vi "DENFPGA.vi"(8 "error in (no error)":errorcluster, 9 "Single shot":bool, 10 "Reads":u8[](array[numeric])=[0, 0, 0, 0, 0, 0, 0, 0, 0, 0, 0, 0, 0, 0, 0, 0, 0, 0, 0, 0, 0, 0, 0, 0, 0, 0, 0, 0, 0, 0, 0, 0, 0, 0, 0, 0, 0, 0, 0, 0, 0, 0, 0, 0, 0, 0, 0, 0, 0, 0, 0, 0, 0, 0, 0, 0, 0, 0, 0, 0, 0, 0, 0, 0, 0, 0, 0, 0, 0, 0, 0, 0, 0, 0, 0, 0, 0, 0, 0, 0, 0, 0, 0, 0, 0, 0, 0, 0, 0, 0, 0, 0, 0, 0, 0, 0, 0, 0, 0, 0], 11 "Commands":u8[](array[numeric])=[0, 0, 0, 0, 0, 0, 0, 0, 0, 0, 0, 0, 0, 0, 0, 0, 0, 0, 0, 0, 0, 0, 0, 0, 0, 0, 0, 0, 0, 0, 0, 0, 0, 0, 0, 0, 0, 0, 0, 0, 0, 0, 0, 0, 0, 0, 0, 0, 0, 0, 0, 0, 0, 0, 0, 0, 0, 0, 0, 0, 0, 0, 0, 0, 0, 0, 0, 0, 0, 0, 0, 0, 0, 0, 0, 0, 0, 0, 0, 0, 0, 0, 0, 0, 0, 0, 0, 0, 0, 0, 0, 0, 0, 0, 0, 0, 0, 0, 0, 0]) -> (0 "error out":errorcluster, 1 "Telemetry":u8[](array[numeric]), 2 "IP on error/exit":i16, 3 "Readouts":u8[](array[numeric]), 4 "code":i32, 5 "status":bool)   [LabVIEW 2018]
uses:
  TestMPU.lvclass
  <vilib>/rvi/Emulation/niFpgaSctlEmulationGetInTimedLoop.vi
  <vilib>/rvi/DataTransferAndStorage/Container/Common/niFpgaContainerGetUniqueNameForEmu.vi
  <vilib>/rvi/DataTransferAndStorage/Container/Common/niFpgaContainerSetEmuInfo.vi
  <vilib>/rvi/eio/common/nirviEmuReportErrorAndStop.vi
  <vilib>/rvi/DataTransferAndStorage/Container/Common/niFpgaContainerExecOnDevCompGetState.vi
  <vilib>/rvi/Emulation/niFpgaEmulationIsFPGAContextNoSignature.vi
  <vilib>/rvi/errors/niFpgaSetErrorForExecOnDevCompSimple.vi
  <vilib>/rvi/FIFO/Fifo_Resource/nirvififoEmulationSetSize.vi
  <vilib>/rvi/FIFO/Fifo_Resource/nirviFifoEmulationQueueMgr.vi
  <instcachedir>/0/nirviFifoEmulationQueueMgr_E5CAEC123FF24DC58D834DCA3CDAA9B5.lvgen/nirviFifoEmulationQueueMgr_E5CAEC123FF24DC58D834DCA3CDAA9B5_001.vi
  <vilib>/rvi/FIFO/Fifo_Resource/nirvififoEmulationDetermineInputValidOut.vi
  <vilib>/rvi/FIFO/Fifo_Resource/nirvififoEmulationCreateLock.vi
  <vilib>/rvi/Emulation/niFpgaProcessEmulError.vi
  <vilib>/rvi/FIFO/Fifo_Resource/nirvififoEmulationObtainLock.vi
  <vilib>/rvi/FIFO/Fifo_Resource/nirvififoEmulationReleaseLock.vi
  <vilib>/rvi/occurrence/nirviWaitOnOccurrenceBase.vi
  <vilib>/rvi/errors/nirviReportUnexpectedCaseInternalError.vi
  <vilib>/rvi/errors/nirviReportUnexpectedCaseInternalError (U32).vi
  <vilib>/Utility/error.llb/Clear Errors.vi
  <vilib>/rvi/interface/RandomDataEmulation/niFpgaRandomDataHandleErrors.vi
  <vilib>/rvi/LocalResourceManager/LocalResourceManager.xnode
  <vilib>/rvi/DataTransferAndStorage/Container/XNode/niFpgaContainer.xnode
  <vilib>/rvi/FIFO/Fifo_Resource/niFpgaFifoEmulationRefIn.vi
panel:
  out "Writes":u8[](array[numeric])
  # "You need to fill in commands. First element of\ncommands is number of commands (same for reads, as \ncommands array is fixed size itself). If number of commands\nis <= 0, error -23 is triggered and execution doesn't proceed."
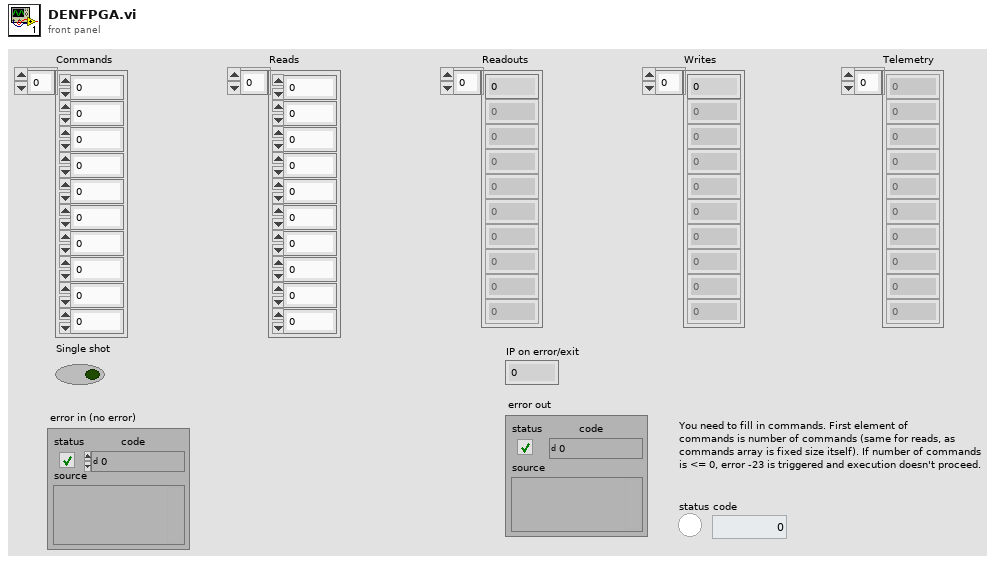
[diagram p1: front panel]
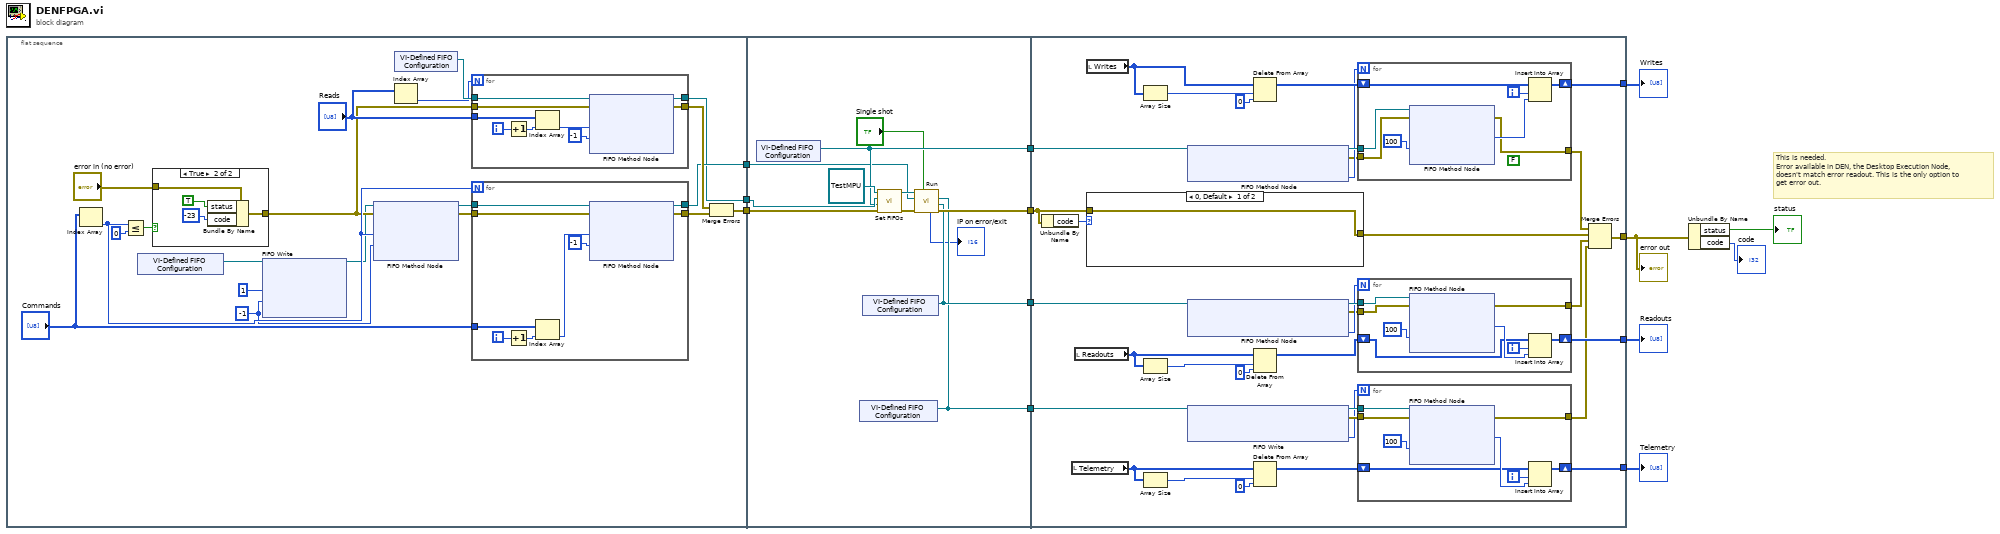
[diagram p0: block diagram]
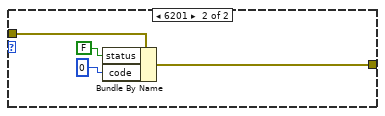
[diagram p3: hidden frame]
diagram:
  # "This is needed.\nError available in DEN, the Desktop Execution Node,\ndoesn't match error readout. This is the only option to \nget error out."
  n1 = flat-sequence {
    tunnel: [w24] -> w13
    tunnel: [w23] -> w12
    tunnel: [w22] -> w11
    tunnel: w13 -> [w66]
    tunnel: w12 -> [w59]
    tunnel: w11 -> [w64]
    tunnel: [w61] -> w10
    tunnel: [w63] -> w7
    tunnel: [w62] -> w6
    tunnel: [w60] -> w5
    tunnel: w10 -> [w87]
    tunnel: [w86] -> w9
    tunnel: [w85] -> w8
    tunnel: w7 -> [w84]
    tunnel: w6 -> [w83]
    tunnel: w5 -> [w79]
    tunnel: [w70] -> w4
    tunnel: [w69] -> w3
    frame #0 {
      w15 = -1 ("Timeout")
      n2 = Index Array(array="Commands") -> (element=w21:u8)  [unwired: 1 in]
      n3 = Less Or Equal?(x=w21, y=u8 0) -> (x <= y?=w19:bool)
      n4 = xnode "VI-Defined FIFO Configuration"() -> ("FIFO Out"=w29:refnum<k21>)
      n5 = case shown="True" w19 {
        tunnel: [w34 w37] -> w17
        tunnel: "error in (no error)" -> [w34 w38]
        frame False {
        }
        frame True {
          n6 = Bundle By Name(cluster=w38, "status"=TRUE, "code"=-23) -> (w37:errorcluster)
        }
      }
      n7 = xnode "FIFO Write"("Element"=u8 1, "Timeout"=w15, "FIFO In"=w29) -> ("FIFO Out"=w16:refnum<k21>)  [unwired: 1 out]
      n8 = xnode ("FIFO Method Node")("Element"=w21, "Timeout"=w15, "error in (no error)"=w17, "FIFO In"=w16) -> ("error out"=w26:errorcluster, "FIFO Out"=w30:refnum<k21>)  [unwired: 1 out]
      n9 = Index Array(array="Reads") -> (element=w27:u8)  [unwired: 1 in]
      n10 = xnode "VI-Defined FIFO Configuration"() -> ("FIFO Out"=w31:refnum<k21>)
      n11 = for {
        N: w27 -> [_]
        tunnel: "Reads" -> [w43]
        tunnel: w31 -> [w41]
        tunnel: [w40] -> w22
        tunnel: w17 -> [w46]
        tunnel: [w39] -> w32
        i -> [w45]
        n12 = Increment(x=w45) -> (x+1=w44:i32)
        n13 = Index Array(array=w43, index=w44) -> (element=w42:u8)
        n14 = xnode ("FIFO Method Node")("Element"=w42, "Timeout"=-1, "error in (no error)"=w46, "FIFO In"=w41) -> ("error out"=w39:errorcluster, "FIFO Out"=w40:refnum<k21>)  [unwired: 1 out]
      }
      n15 = for {
        N: w21 -> [_]
        tunnel: "Commands" -> [w56]
        tunnel: w30 -> [w50]
        tunnel: [w49] -> w23
        tunnel: w26 -> [w52]
        tunnel: [w48] -> w33
        i -> [w55]
        n16 = Increment(x=w55) -> (x+1=w54:i32)
        n17 = Index Array(array=w56, index=w54) -> (element=w53:u8)
        n18 = xnode ("FIFO Method Node")("Element"=w53, "Timeout"=-1, "error in (no error)"=w52, "FIFO In"=w50) -> ("error out"=w48:errorcluster, "FIFO Out"=w49:refnum<k21>)  [unwired: 1 out]
      }
      n19 = Merge Errors(w32, w33) -> (w24:errorcluster)
    }
    frame #1 {
      n20 = xnode "VI-Defined FIFO Configuration"() -> ("FIFO Out"=w62:refnum<k21>)
      n21 = xnode "VI-Defined FIFO Configuration"() -> ("FIFO Out"=w60:refnum<k21>)
      n22 = xnode "VI-Defined FIFO Configuration"() -> ("FIFO Out"=w61:refnum<k21>)
      n23 = call-dynamic "Set FIFOs.vi"("error in (no error)"=w66, "Output"=w62, "Input"=w64, "TestMPU in"=refnum<class "TestMPU.lvclass"> refnum ("TestMPU.lvclass")) -> ("error out"=w67:errorcluster, "TestMPU out"=w68:refnum<class "TestMPU.lvclass">)  [unwired: 6 in]
      n24 = call-dynamic "Run.vi"("DebugOut"=w61, "Telemetry"=w60, "Exit on end"="Single shot", "error in (no error)"=w67, "Command FIFO"=w59, "MPU in"=w68) -> ("error out"=w63:errorcluster, "IP On Error"=→"IP on error/exit":i16)  [unwired: 3 in, 1 out]
    }
    frame #2 {
      n25 = Unbundle By Name(w84) -> ("code"=w94:i32)
      n26 = local read "Telemetry"() -> (w71:u8[])
      n27 = local read "Readouts"() -> (w100:u8[])
      n28 = local read "Writes"() -> (w96:u8[])
      n29 = case shown="0, Default" w94 {
        tunnel: [w111 w114] -> w81
        tunnel: w84 -> [w111 w115]
        frame 0, Default {
        }
        frame 6201 {
          n30 = Bundle By Name(cluster=w115, "status"=FALSE, "code"=0) -> (w114:errorcluster)
        }
      }
      n31 = Array Size(array=w96) -> (size(s)=w97:i32)
      n32 = Array Size(array=w100) -> (size(s)=w98:i32)
      n33 = Array Size(array=w71) -> (size(s)=w78:i32)
      n34 = xnode ("FIFO Method Node")("FIFO In"=w83) -> ("Number of Elements to Read"=w91:u32, "error out"=w90:errorcluster, "FIFO Out"=w102:refnum<k21>)  [unwired: 1 in]
      n35 = xnode ("FIFO Method Node")("FIFO In"=w87) -> ("Number of Elements to Read"=w93:u32, "error out"=w92:errorcluster, "FIFO Out"=w101:refnum<k21>)  [unwired: 1 in]
      n36 = xnode "FIFO Write"("FIFO In"=w79) -> ("Number of Elements to Read"=w72:u32, "error out"=w75:errorcluster, "FIFO Out"=w76:refnum<k21>)  [unwired: 1 in]
      n37 = Delete From Array(array=w96, length=w97, index=0) -> (array with subset deleted=w95:u8[])  [unwired: 1 out]
      n38 = Delete From Array(array=w100, length=w98, index=0) -> (array with subset deleted=w99:u8[])  [unwired: 1 out]
      n39 = Delete From Array(array=w71, length=w78, index=0) -> (array with subset deleted=w73:u8[])  [unwired: 1 out]
      n40 = for {
        N: w91 -> [_]
        shift-right: [w127] -> w85
        shift-left: w95 -> [w128]
        tunnel: w102 -> [w125]
        tunnel: w90 -> [w126]
        tunnel: [w124] -> w80
        i -> [w129]
        (unwired) FALSE
        n41 = xnode ("FIFO Method Node")("Timeout"=100, "error in (no error)"=w126, "FIFO In"=w125) -> ("Element"=w130:u8, "error out"=w124:errorcluster)  [unwired: 2 out]
        n42 = Insert Into Array(array=w128, index=w129, new element=w130) -> (w127:u8[])
      }
      n43 = for {
        N: w93 -> [_]
        shift-right: [w120] -> w86
        shift-left: w99 -> [w118]
        tunnel: w101 -> [w117]
        tunnel: w92 -> [w123]
        tunnel: [w116] -> w82
        i -> [w119]
        n44 = xnode ("FIFO Method Node")("Timeout"=100, "error in (no error)"=w123, "FIFO In"=w117) -> ("Element"=w122:u8, "error out"=w116:errorcluster)  [unwired: 2 out]
        n45 = Insert Into Array(array=w118, index=w119, new element=w122) -> (w120:u8[])
      }
      n46 = for {
        N: w72 -> [_]
        shift-right: [w107] -> w70
        shift-left: w73 -> [w105]
        tunnel: w76 -> [w104]
        tunnel: w75 -> [w110]
        tunnel: [w103] -> w74
        i -> [w106]
        n47 = xnode ("FIFO Method Node")("Timeout"=100, "error in (no error)"=w110, "FIFO In"=w104) -> ("Element"=w109:u8, "error out"=w103:errorcluster)  [unwired: 2 out]
        n48 = Insert Into Array(array=w105, index=w106, new element=w109) -> (w107:u8[])
      }
      n49 = Merge Errors(w80, w81, w82, w74) -> (w69:errorcluster)
    }
  }
  n50 = Unbundle By Name(w3) -> ("status"=→"status":bool, "code"=→"code":i32)
  "Writes" <- w8
  "Readouts" <- w9
  "Telemetry" <- w4
  "error out" <- w3
